vi "gc-zyklus mfc mpos.vi"() -> ()   [LabVIEW 2010]
uses:
  <vilib>/Instr/_visa.llb/VISA Configure Serial Port (Instr).vi
panel:
  out "Zeitpunkt":string
  out "Temperatur (°C)":u16
  out "Meßwert PC2 (mbara)":u16
  out "Meßwert PC1 (mbara)":u16
  out "Meßwert FC (mln/min)":u16
  in  "Setpoint PC1 (bara)":dbl min=0.15 max=3.0 step=0.05
  in  "Setpoint PC2 (bara)":dbl min=0.15 max=3.0 step=0.05
  in  "Dateipfad (Dialog verwenden)":path
  out "Zyklus Nr.":i32
  in  "Positionen (1-6)":i32[](array[numeric])=[1, 3, 5, 2]
  out "Anzahl der Zustände (Mpos.-Ventil)":i32
  out "Position":i32
  in  "Setpoints FC (ln/min)":dbl[](array[numeric])=[1.0, 3.0, 5.0, 2.0]
  in  "Längen der Zustände (s)":i32[](array[numeric])=[1, 3, 5, 2]
  out "Anzahl der Zustände (MFC)":i32
  out "Länge des Zustandes \"i\" (s)":i32
  out "Setpoint \"i\" FC (ln/min)":dbl
  out "Sequenz Nr.":i32
  out "Aktuelle Zeit":timestamp
  in  "(Sequenz wird zu Ende geführt)":bool
  # "Gerät im Chromatographie-Zyklus, z.B. MFC"
  # "Multipositionsventil"
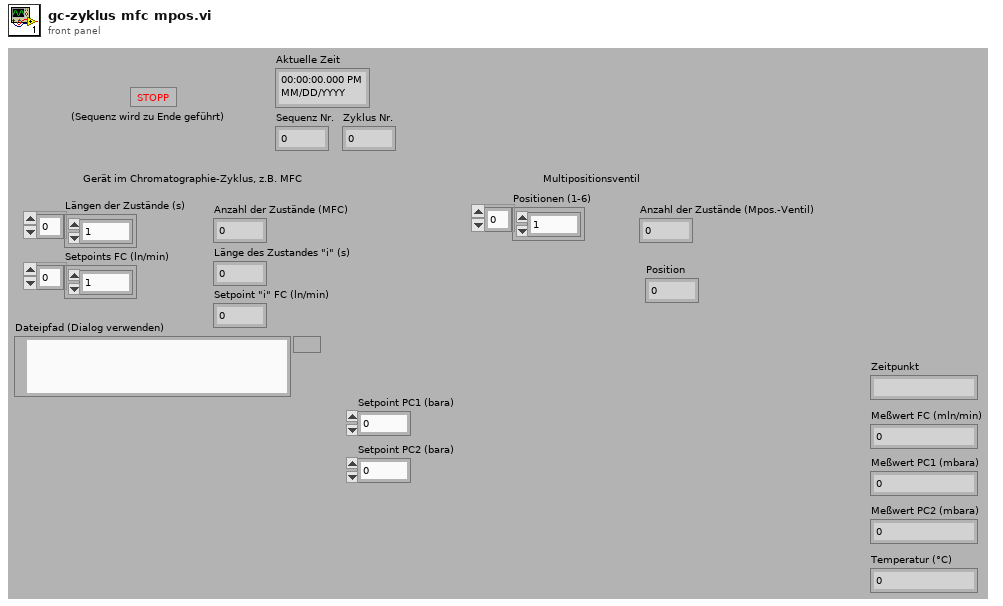
[diagram p1: front panel]
types:
  T1 = enum16{"open", "replace", "create", "open or create", "replace or create", "replace or create with confirmation"}
  T2 = cluster{"Mode":enum16{"RTU", "ASCII"}, "Slave Address":u8}
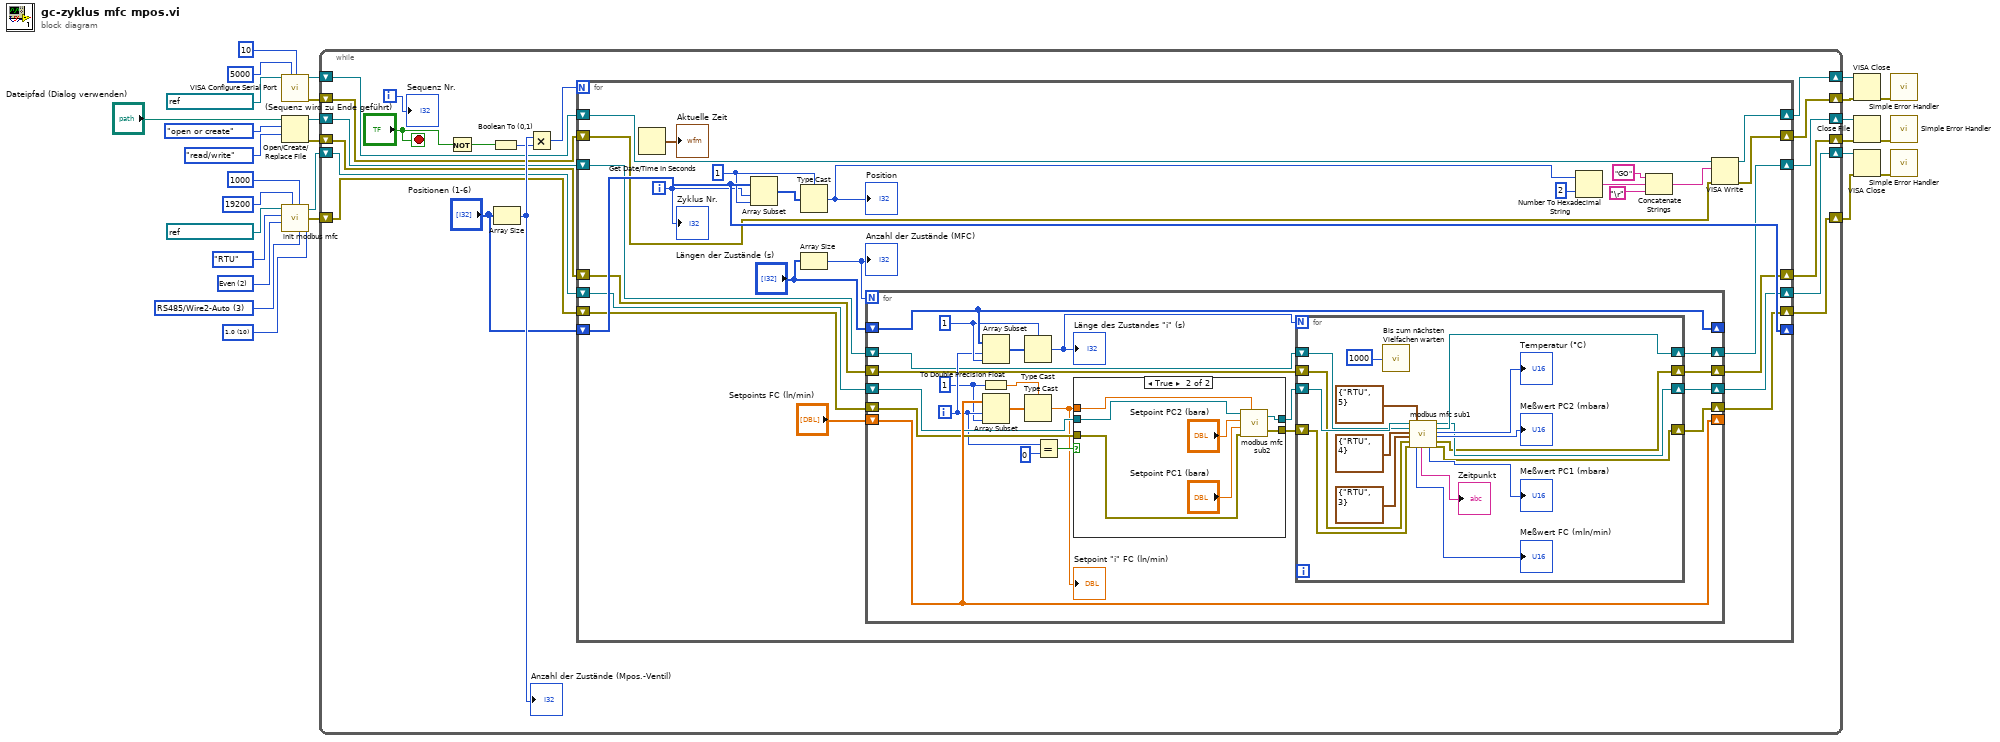
[diagram p0: block diagram]
diagram:
  w25 = u16 10 items=["1.0"=10, "1.5"=15, "2.0"=20] ("Serial Settings:Stop Bits")
  w23 = u16 2 items=["None", "Odd", "Even", "Mark", "Space"] ("Parity")
  w24 = i16 3 items=["Unknown"=-1, "RS485/Wire4"=0, "RS485/Wire2-EchoDTR"=1, "RS485/Wire2-CtrlDTR"=2, "RS485/Wire2-Auto"=3, "RS232/DTE"=128, "RS232/DCE"=129, "RS232/AUTO"=130] ("Serial Settings:Wire Mode")
  n1 = call-poly "VISA Configure Serial Port"("VISA resource name"=refnum<visa-resource-name> "ASRL1::INSTR", "timeout (10sec)"=u32 5000, "termination char\n(0xA = '\\n' = LF)"=u8 10 ("termination char\n(0xA = '\\n' = LF)")) -> ("VISA resource name out"=w5:refnum<visa-resource-name>, "error out"=w4:errorcluster)  [unwired: 11 in]
  n2 = Open/Create/Replace File(file path (use dialog)="Dateipfad (Dialog verwenden)", operation (0:open)=T1."open or create" ("Operation (0:Öffnen)"), access (0:read/write)=enum16{"read/write", "read-only", "write-only"}."read/write" ("Zugriff (0:Lesen/Schreiben)")) -> (refnum out=w18:refnum<file>, error out=w17:errorcluster)  [unwired: 3 in, 1 out]
  n3 = call "init modbus mfc.vi"("Timeout"=u32 1000, "Serial Settings:Stop Bits"=w25, "Serial Settings:Wire Mode"=w24, "Baud Rate"=u32 19200, "VISA resource name"=refnum<visa-resource-name> "ASRL2::INSTR", "Mode"=enum16{"RTU", "ASCII"}."RTU", "Parity"=w23) -> ("VISA resource name out"=w16:refnum<visa-resource-name>, "error out"=w15:errorcluster)  [unwired: 2 in]
  n4 = while {
    shift-right: [w36] -> w9
    shift-left: w18 -> [w40]
    shift-right: [w35] -> w8
    shift-left: w17 -> [w39]
    shift-right: [w34] -> w7
    shift-left: w16 -> [w38]
    shift-right: [w33] -> w6
    shift-left: w15 -> [w37]
    shift-right: [w30] -> w2
    shift-left: w5 -> [w32]
    shift-right: [w29] -> w1
    shift-left: w4 -> [w31]
    i -> [w47]
    stop <- "(Sequenz wird zu Ende geführt)" stop-if-true
    n5 = Not(x="(Sequenz wird zu Ende geführt)") -> (.not. x?=w44:bool)
    n6 = Boolean To (0,1)(Boolean=w44) -> (0, 1=w42:i16)
    n7 = Array Size(array="Positionen (1-6)") -> (size(s)=w46:i32)
    "Anzahl der Zustände (Mpos.-Ventil)" <- w46
    n8 = Multiply(x=w46, y=w42) -> (x*y=w43:i32)
    n9 = for {
      N: w43 -> [_]
      shift-right: [w73] -> _
      shift-left: "Positionen (1-6)" -> [w73]
      shift-right: [w55] -> w36
      shift-left: w40 -> [w63]
      shift-right: [w54] -> w35
      shift-left: w39 -> [w64]
      shift-right: [w53] -> w34
      shift-left: w38 -> [w66]
      shift-right: [w52] -> w33
      shift-left: w37 -> [w65]
      shift-right: [w49] -> w30
      shift-left: w32 -> [w51]
      shift-right: [w48] -> w29
      shift-left: w31 -> [w50]
      i -> [w70]
      w72 = 1 ("Länge")
      n10 = Get Date/Time In Seconds() -> (seconds since 1Jan1904=→"Aktuelle Zeit":timestamp)
      n11 = Array Subset(array=w73, index=w70, length=w72) -> (w71:i32[])
      n12 = Type Cast(type=w72, x=w71) -> (*(type *) &x=w56:i32)
      "Position" <- w56
      n13 = Array Size(array="Längen der Zustände (s)") -> (size(s)=w62:i32)
      "Anzahl der Zustände (MFC)" <- w62
      n14 = for {
        N: w62 -> [_]
        shift-right: [w95] -> _
        shift-left: "Längen der Zustände (s)" -> [w95]
        shift-right: [w91] -> _
        shift-left: "Setpoints FC (ln/min)" -> [w91]
        shift-right: [w78] -> w55
        shift-left: w63 -> [w79]
        shift-right: [w76] -> w54
        shift-left: w64 -> [w80]
        shift-right: [w77] -> w53
        shift-left: w66 -> [w90]
        shift-right: [w75] -> w52
        shift-left: w65 -> [w89]
        i -> [w88]
        w84 = 1 ("Länge")
        w94 = 1 ("Länge")
        n15 = Array Subset(array=w95, index=w88, length=w94) -> (w93:i32[])
        n16 = To Double Precision Float(number=w84) -> (double precision float=w83:dbl)
        n17 = Array Subset(array=w91, index=w88, length=w84) -> (w92:dbl[])
        n18 = Type Cast(type=w94, x=w93) -> (*(type *) &x=w85:i32)
        "Länge des Zustandes \"i\" (s)" <- w85
        n19 = Type Cast(type=w83, x=w92) -> (*(type *) &x=w74:dbl)
        "Setpoint \"i\" FC (ln/min)" <- w74
        n20 = Equal?(x=w88, y=0) -> (x = y?=w86:bool)
        n21 = case shown="True" w86 {
          tunnel: w89 -> [w114 w120]
          tunnel: [w114 w119] -> w82
          tunnel: w90 -> [w113 w121]
          tunnel: [w113 w118] -> w81
          tunnel: w74 -> [_ w115]
          frame False {
          }
          frame True {
            n22 = call "modbus mfc sub2.vi"("VISA resource name out 2"=w121, "Setpoint PC2 (bara)"="Setpoint PC2 (bara)", "Setpoint PC1 (bara)"="Setpoint PC1 (bara)", "error out 2"=w120, "Setpoint FC (ln/min)"=w115) -> ("VISA resource name out"=w118:refnum<visa-resource-name>, "error out"=w119:errorcluster)
          }
        }
        n23 = for {
          N: w85 -> [_]
          shift-right: [w98] -> w77
          shift-left: w81 -> [w102]
          shift-right: [w99] -> w78
          shift-left: w79 -> [w100]
          shift-right: [w97] -> w76
          shift-left: w80 -> [w101]
          shift-right: [w96] -> w75
          shift-left: w82 -> [w103]
          n24 = call "Bis zum nächsten Vielfachen warten"("Count(mSec)"=u32 1000) -> ()  [unwired: 1 out]
          n25 = call "modbus mfc sub1.vi"("VISA resource name out"=w102, "refnum out 2"=w100, "Serial Parameters 2"=T2 {"Mode"=enum."RTU", "Slave Address"=4}, "Serial Parameters"=T2 {"Mode"=enum."RTU", "Slave Address"=3}, "error out 2"=w101, "error out 3"=w103, "Serial Parameters 3"=T2 {"Mode"=enum."RTU", "Slave Address"=5}) -> ("Numerisch 3"=→"Meßwert FC (mln/min)":u16, "date/time string"=→"Zeitpunkt":string, "Numerisch 2"=→"Meßwert PC1 (mbara)":u16, "VISA resource name out 2"=w98:refnum<visa-resource-name>, "refnum out"=w99:refnum<file>, "Numerisch 4"=→"Temperatur (°C)":u16, "Numerisch"=→"Meßwert PC2 (mbara)":u16, "error out"=w97:errorcluster, "error out 4"=w96:errorcluster)  [unwired: 3 in, 1 out]
        }
      }
      n26 = Number To Hexadecimal String(1:i16 2 ("Breite (-)"), 2:w56) -> (0:w60:string)
      n27 = Concatenate Strings("GO" ("String"), w60, "\r") -> (w61:string)
      n28 = VISA Write(VISA resource name=w51, write buffer=w61, error in (no error)=w50) -> (VISA resource name out=w49:refnum<visa-resource-name>, error out=w48:errorcluster)  [unwired: 1 out]
      "Zyklus Nr." <- w70
    }
    "Sequenz Nr." <- w47
  }
  n29 = VISA Close(VISA resource name=w2, error in (no error)=w1) -> (error out=w3:errorcluster)
  n30 = Close File(refnum=w9, error in=w8) -> (error out=w13:errorcluster)  [unwired: 1 out]
  n31 = VISA Close(VISA resource name=w7, error in (no error)=w6) -> (error out=w14:errorcluster)
  n32 = call <vilib>:"Simple Error Handler.vi"("error in (no error)"=w3) -> ()  [unwired: 4 in, 5 out]
  n33 = call <vilib>:"Simple Error Handler.vi"("error in (no error)"=w13) -> ()  [unwired: 4 in, 5 out]
  n34 = call <vilib>:"Simple Error Handler.vi"("error in (no error)"=w14) -> ()  [unwired: 4 in, 5 out]
